vi "crio_9073_dual_motor_plant.vi"() -> ()   [LabVIEW 2019]
uses:
  <vilib>/rvi/Analysis/control/PID/Typedef/niFpgaPID_ManualControl.ctl
  <vilib>/FPGAPlugInAG/cRIO-9073/niLvFpga_Open_cRIO-9073.vi
  <vilib>/rvi/interface/common/dynamic/niFpgaDynamicAddResources.vi
  <vilib>/Utility/error.llb/Error Cluster From Error Code.vi
  <vilib>/rvi/errors/niLvFpgaAdjustHostInterfaceError.vi
  <vilib>/FPGAPlugInAG/Dynamic/niLvFpga_Close_Dynamic.vi
  <vilib>/rvi/interface/nirviOpenFPGA/nirviOpenFPGA.xnode
  On Call Bitfiles/gpass2_FPGATarget3_crioFPGAPlantDua_oyerNF4c0pQ.lvbitx
  <vilib>/rvi/interface/nirviReadWriteControl/nirviReadWriteControl.xnode
  <vilib>/rvi/interface/nirviCloseFPGA/nirviCloseFPGA.xnode
  <vilib>/rvi/interface/Simulation/niFpgaSimulationCallBeginRW.vi
  NiFpgaLv.dll
panel:
  in  "manual control load":T1 {"manual input (0)" scale=-1.0..1.0}
  in  "manual control":T1 {"manual input (0)" scale=-1.0..1.0}
  out "Velocity (Counts/Interval) Load":i32
  in  "stop":bool
  out "Position (Counts) Load":i64
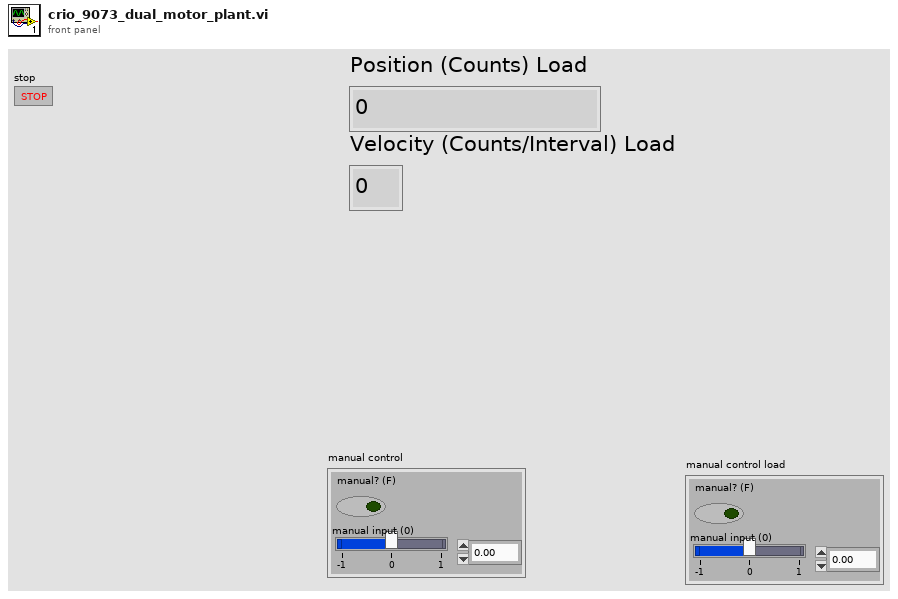
[diagram p1: front panel]
types:
  T1 = typedef "niFpgaPID_ManualControl.ctl" = cluster{"manual? (F)":bool, "manual input (0)":sgl}
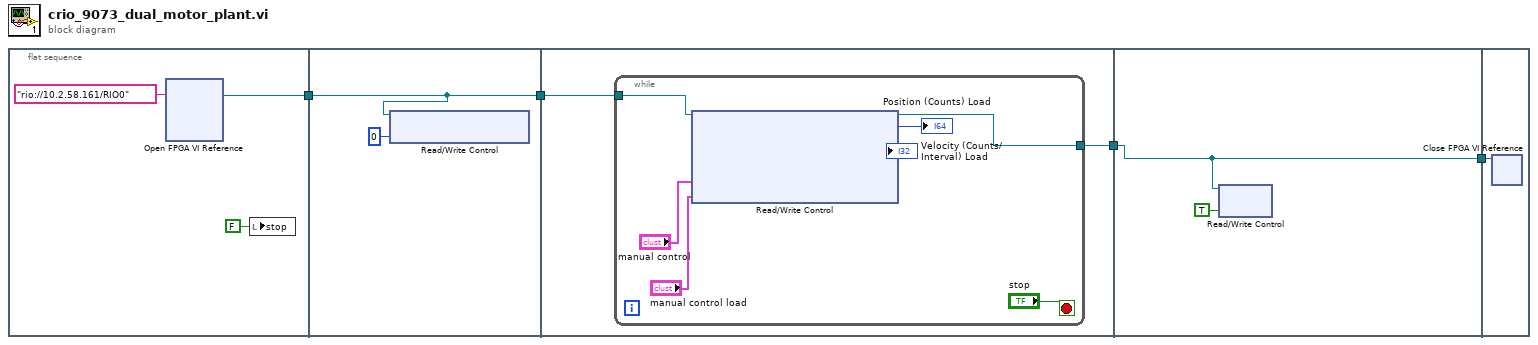
[diagram p0: block diagram]
diagram:
  n1 = flat-sequence {
    tunnel: [w6] -> w3
    tunnel: w3 -> [w9]
    tunnel: [w9] -> w2
    tunnel: w2 -> [w11]
    tunnel: [w10] -> w4
    tunnel: w4 -> [w20]
    tunnel: [w20] -> w1
    tunnel: w1 -> [w21]
    frame #0 {
      n2 = xnode "Open FPGA VI Reference"("resource name"=tag "rio://10.2.58.161/RIO0") -> ("FPGA VI Reference Out"=w6:refnum<k20>)  [unwired: 1 in, 1 out]
      n3 = local write "stop"(FALSE ("stop")) -> ()
    }
    frame #1 {
      n4 = xnode "Read/Write Control"("FPGA VI Reference In"=w9, "Position (Counts) Load"=i64 0) -> ()  [unwired: 1 in, 2 out]
    }
    frame #2 {
      n5 = while {
        tunnel: w11 -> [w18]
        tunnel: [w15] -> w10
        stop <- "stop" stop-if-true
        n6 = xnode "Read/Write Control"("FPGA VI Reference In"=w18, "manual control"="manual control", "manual control Load"="manual control load") -> ("FPGA VI Reference Out"=w15:refnum<k20>, "Position (Counts) Load"=→"Position (Counts) Load":i64, "Velocity (Counts/Interval) Load"=→"Velocity (Counts/Interval) Load":i32)  [unwired: 1 in, 2 out]
      }
    }
    frame #3 {
      n7 = xnode "Read/Write Control"("FPGA VI Reference In"=w20, "stop"=TRUE) -> ()  [unwired: 1 in, 2 out]
    }
    frame #4 {
      n8 = xnode "Close FPGA VI Reference"("FPGA VI Reference In"=w21) -> ()  [unwired: 1 in, 1 out]
    }
  }
